vi "End Tasks.vi"(1 "AO Task In":refnum<k21>[](array[refnum])=[""], 2 "AI Task In":refnum<k21>[](array[refnum])=["", ""]) -> ()   [LabVIEW 2011, in "Lock-In Variable Channels_2.lvclass"]
uses:
  Lock-In Variable Channels_2.lvclass
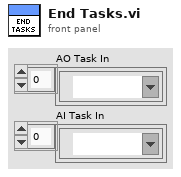
[diagram p1: front panel]
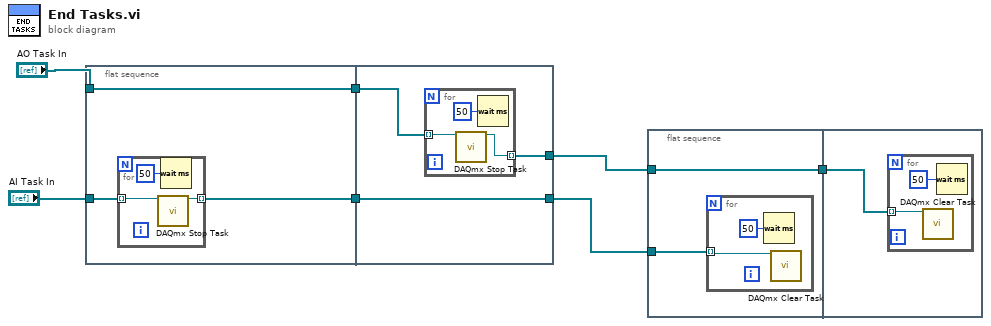
[diagram p0: block diagram]
diagram:
  n1 = flat-sequence {
    tunnel: "AI Task In" -> [w10]
    tunnel: [w9] -> w7
    tunnel: "AO Task In" -> [w9]
    tunnel: [w8] -> w6
    tunnel: w7 -> [w16]
    tunnel: w6 -> [w15]
    tunnel: [w15] -> w3
    tunnel: [w14] -> w4
    frame #0 {
      n2 = for {
        tunnel: w10 -> [w13] mode=indexing
        tunnel: [w11] -> w8 mode=indexing
        n3 = call <vilib>:"DAQmx Stop Task.vi"("task/channels in"=w13) -> ("task out"=w11:refnum<k21>)  [unwired: 13 in, 1 out]
        n4 = Wait (ms)(milliseconds to wait=u32 50) -> ()  [unwired: 1 out]
      }
    }
    frame #1 {
      n5 = for {
        tunnel: w16 -> [w19] mode=indexing
        tunnel: [w17] -> w14 mode=indexing
        n6 = call <vilib>:"DAQmx Stop Task.vi"("task/channels in"=w19) -> ("task out"=w17:refnum<k21>)  [unwired: 13 in, 1 out]
        n7 = Wait (ms)(milliseconds to wait=u32 50) -> ()  [unwired: 1 out]
      }
    }
  }
  n8 = flat-sequence {
    tunnel: w3 -> [w21]
    tunnel: w4 -> [w20]
    tunnel: [w20] -> w5
    tunnel: w5 -> [w24]
    frame #0 {
      n9 = for {
        tunnel: w21 -> [w23] mode=indexing
        n10 = Wait (ms)(milliseconds to wait=u32 50) -> ()  [unwired: 1 out]
        n11 = call <vilib>:"DAQmx Clear Task.vi"("task in"=w23) -> ()  [unwired: 14 in, 1 out]
      }
    }
    frame #1 {
      n12 = for {
        tunnel: w24 -> [w26] mode=indexing
        n13 = call <vilib>:"DAQmx Clear Task.vi"("task in"=w26) -> ()  [unwired: 14 in, 1 out]
        n14 = Wait (ms)(milliseconds to wait=u32 50) -> ()  [unwired: 1 out]
      }
    }
  }
